vi "W22B.vi"(1 "Parallel Word In":bool[][](array[boolean]), 2 "Bits-per-Symbol":i32, 3 "Number of Subcarries":i32) -> (0 "Parallel Output":bool[](array[boolean]))   [LabVIEW 2013]
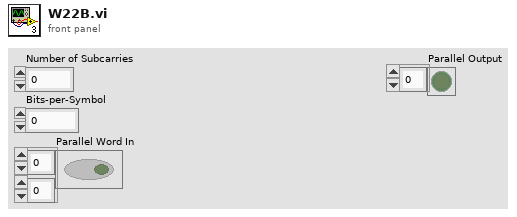
[diagram p1: front panel]
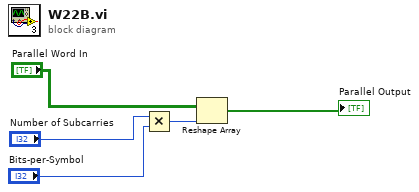
[diagram p0: block diagram]
diagram:
  n1 = Multiply(x="Number of Subcarries", y="Bits-per-Symbol") -> (x*y=w3:i32)
  n2 = Reshape Array("Parallel Word In", w3) -> (→"Parallel Output":bool[])
